vi "Configure_Interrupt_Source.vi"(7 "I2C Channel":u8, 8 "error in":errorcluster, 9 "INT<n> Configuration":T1 {"Advanced" items=["OR Combination of Interrupts"=0, "6 Direction Movement Recognition"=64, "AND Combination of Interrupts"=128, "6 Direction Position Recognition"=192]; "Advenced" items=["Z> Threshold INT DISABLE"=0, "Z> Threshold INT ENABLE"=32]; "Advenced 2" items=["Z< Threshold INT DISABLE"=0, "Z< Threshold INT ENABLE"=16]; "Advenced 3" items=["Y> Threshold INT DISABLE"=0, "Y> Threshold INT ENABLE"=8]; "Advenced 4" items=["Y< Threshold INT DISABLE"=0, "Y< Threshold INT ENABLE"=4]; "Advenced 5" items=["X> Threshold INT DISABLE"=0, "X> Threshold INT ENABLE"=2]; "Advenced 6" items=["X< Threshold INT DISABLE", "X< Threshold INT ENABLE"]}, 10 "Interrupt Source":T2(ring), 11 "LINX Resource In":T3) -> (0 "error out":errorcluster, 3 "LINX Resource Out":T3)   [LabVIEW 2014, in "LMH-LINX.lvlib" / "LIS331HH.lvlib"]
uses:
  <vilib>/MakerHub/LINX/Public/Sensors/Accelerometer/LIS331HH/LIS331HH.lvlib
  <vilib>/MakerHub/LINX/Private/Type Defs/LINX Ref.ctl
  <vilib>/MakerHub/LINX/Private/Type Defs/Platform.ctl
  <vilib>/MakerHub/LINX/Private/Type Defs/Interface.ctl
  <vilib>/MakerHub/LINX/Private/Device/Type Defs/LINX Device Config.ctl
  <vilib>/MakerHub/LINX/Private/Device/Type Defs/TCP Config.ctl
  <vilib>/MakerHub/LINX/Private/Device/Type Defs/Channels.ctl
  <vilib>/MakerHub/LINX/Private/Local IO/LinxI2cWrite.vi
  <vilib>/MakerHub/LINX/Public/Utilities/Check Channel.vi
  <vilib>/MakerHub/LINX/Private/Utilties/Generate Error.vi
  <vilib>/MakerHub/LINX/LMH-LINX.lvlib
  <vilib>/MakerHub/LINX/Private/Device/Device.lvlib
panel:
  # "INPUTS"
  # "OUTPUTS"
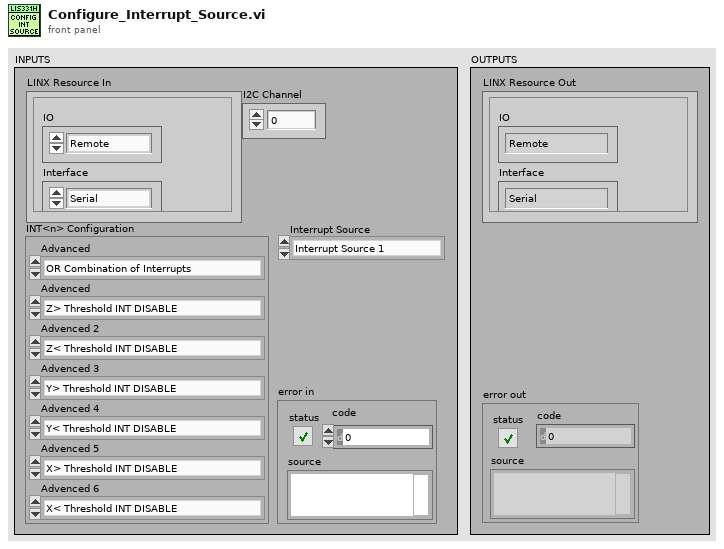
[diagram p1: front panel]
types:
  T1 = cluster{"Advanced":u8, "Advenced":u8, "Advenced 2":u8, "Advenced 3":u8, "Advenced 4":u8, "Advenced 5":u8, "Advenced 6":u8}
  T2 = enum16{"Interrupt Source 1", "Interrupt Source 2"}
  T3 = typedef "LMH-LINX.lvlib/LINX Ref.ctl" = cluster{"IO":T4, "Interface":T5, "LINX Device Config":T6}
  T4 = typedef "LMH-LINX.lvlib/Platform.ctl" = enum16{"Remote", "Local"}
  T5 = typedef "LMH-LINX.lvlib/Interface.ctl" = enum16{"Serial", "TCP"}
  T6 = typedef "LMH-LINX.lvlib/Device.lvlib/LINX Device Config.ctl" = cluster{"Interface":T5, "COM Port":refnum<visa-resource-name>, "TCP Configuration":T7, "Device Family":u8, "Device ID":u8, "Device Name":string, "TCP Ref":refnum<k5>, "Channels":T8}
  T7 = typedef "LMH-LINX.lvlib/Device.lvlib/TCP Config.ctl" = cluster{"IP Address":string, "Port":u16}
  T8 = typedef "LMH-LINX.lvlib/Channels.ctl" = cluster{"DI":u8[], "DO":u8[], "AI":u8[], "AO":u8[], "PWM":u8[], "QE":u8[], "UART":u8[], "I2C 2":u8[], "SPI":u8[], "CAN":u8[], "Servo":u8[], "AI Ref (V)":dbl, "AI Resolution (Bits)":u8, "AO Ref (V)":dbl, "AO Resolution (Bits)":u8}
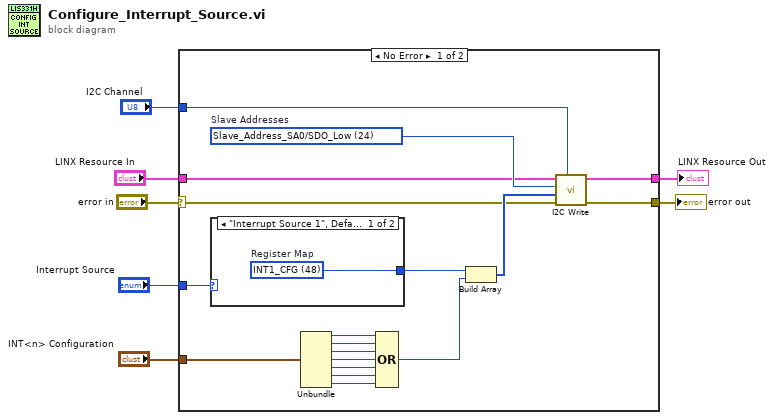
[diagram p0: block diagram]
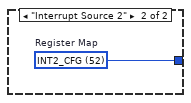
[diagram p2: hidden frame]
diagram:
  n1 = case shown="No Error" "error in" {
    selector: "error in" -> [w17 w29]
    tunnel: [w23 w29] -> w6
    tunnel: "LINX Resource In" -> [w18 w28]
    tunnel: "I2C Channel" -> [w21 _]
    tunnel: [w24 w28] -> w3
    tunnel: "Interrupt Source" -> [w19 _]
    tunnel: "INT<n> Configuration" -> [w16 _]
    frame No Error {
      w22 = u8 24 items=["Slave_Address_SA0/SDO_Low"=24, "Slave_Address_SA0/SDO_High"=25]  # Slave Addresses
      n2 = case shown="\"Interrupt Source 1\", Default" w19 {
        tunnel: [w26 w27] -> w20
        frame "Interrupt Source 1", Default {
          w26 = u8 48 items=["CTRL_REG1"=32, "CTRL_REG2"=33, "CTRL_REG3"=34, "CTRL_REG4"=35, "CTRL_REG5"=36, "HP_FILTER_RESET"=37, "REFERENCE"=38, "STATUS_REG"=39, "OUT_X_L"=40, "OUT_X_H"=41, "OUT_Y_L"=42, "OUT_Y_H"=43, "OUT_Z_L"=44, "OUT_Z_H"=45, "INT1_CFG"=48, "INT1_SOURCE"=49, "INT1_THS"=50, "INT1_DURATION"=51, "INT2_CFG"=52, "INT2_SOURCE"=53, "INT2_THS"=54, "INT2_DURATION"=55]  # Register Map
        }
        frame "Interrupt Source 2" {
          w27 = u8 52 items=["CTRL_REG1"=32, "CTRL_REG2"=33, "CTRL_REG3"=34, "CTRL_REG4"=35, "CTRL_REG5"=36, "HP_FILTER_RESET"=37, "REFERENCE"=38, "STATUS_REG"=39, "OUT_X_L"=40, "OUT_X_H"=41, "OUT_Y_L"=42, "OUT_Y_H"=43, "OUT_Z_L"=44, "OUT_Z_H"=45, "INT1_CFG"=48, "INT1_SOURCE"=49, "INT1_THS"=50, "INT1_DURATION"=51, "INT2_CFG"=52, "INT2_SOURCE"=53, "INT2_THS"=54, "INT2_DURATION"=55]  # Register Map
        }
      }
      n3 = Unbundle(w16) -> ("Advanced"=w15:u8, "Advenced"=w14:u8, "Advenced 2"=w13:u8, "Advenced 3"=w12:u8, "Advenced 4"=w11:u8, "Advenced 5"=w10:u8, "Advenced 6"=w9:u8)
      n4 = Compound Arithmetic op=OR(w15, w14, w13, w12, w11, w10, w9) -> (w8:u8)
      n5 = Build Array(w20, w8) -> (w25:u8[])
      n6 = call <vilib>:"I2C Write.vi"("I2C Channel"=w21, "Error In"=w17, "Data"=w25, "I2C Slave Address (0)"=w22, "LINX Resource"=w18) -> ("Error Out"=w23:errorcluster, "LINX Resource"=w24:T3)  [unwired: 5 in]
    }
    frame Error {
    }
  }
  "error out" <- w6
  "LINX Resource Out" <- w3
